vi "scanclass_1ms_10dt.vi"() -> (0 "max jitter (uS)":dbl format="%.2f", 1 "mean time (uS)":dbl format="%.2f", 2 "standard deviation (uS)":dbl format="%.2f", 3 "execution histogram":T1(graph), 4 "Error":errorcluster, 5 "execution times (uS)":dbl[](graph))   [LabVIEW 2013]
uses:
  scan engine timing source/scan engine timing source.lvclass
  scan engine timing source/scan engine timing source.lvclass/scan engine timing source.ctl
  <vilib>/Platform/TimedLoop/XDataNode/timing_clust.ctl
  <vilib>/Platform/TimedLoop/XDataNode/nitl_modes.ctl
  <vilib>/Platform/TimedLoop/XDataNode/wakeup.ctl
  scan engine timing source/Write scan period (uSec).vi
  <vilib>/platform/TimedLoop/XDataNode/XDataNode.xnode
  <vilib>/Platform/TimedLoop/XDataNode/XDNodeRunTimeDep.lvlib
  <vilib>/NI_Real-Time Target Support.lvlib
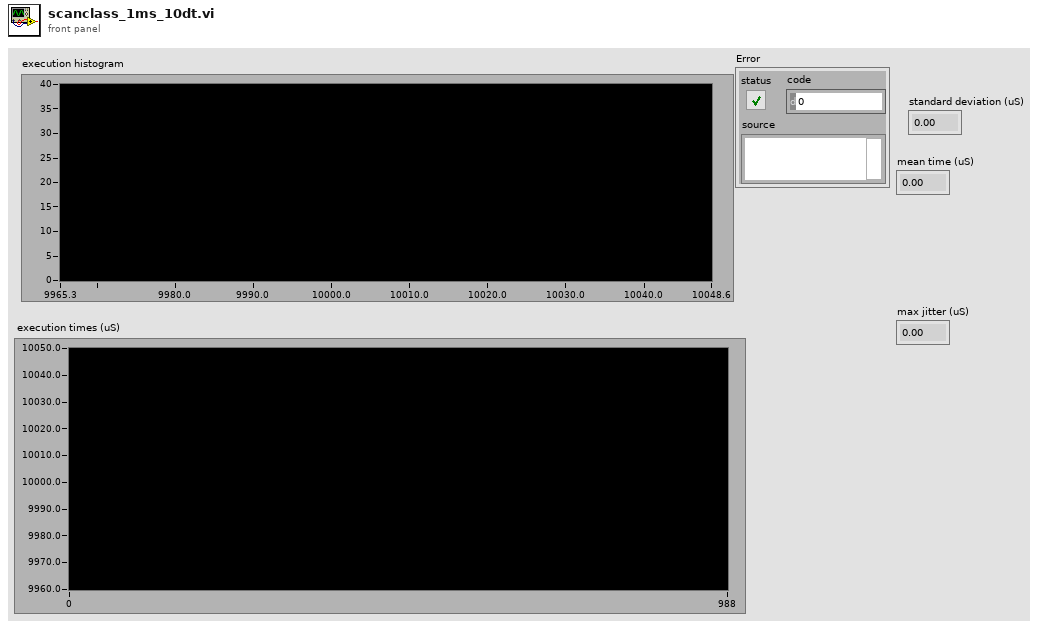
[diagram p1: front panel]
types:
  T1 = cluster{"X Values":dbl[], "Histogram: h(x)":i32[]}
  T2 = typedef "XDNodeRunTimeDep.lvlib/timing_clust.ctl" = cluster{"Expected End [f-1]":u64, "Actual End [f-1]":u64, "Finished Late? [f-1]":bool, "Expected End [i-1]":u64, "Actual End [i-1]":u64, "Finished Late? [i-1]":bool, "Expected Start [i]":u64, "Actual Start [i]":u64, "Expected Start [f]":u64, "Actual Start [f]":u64, "Source Name":string, "Structure Name":string, "Period":i64, "Deadline":i64, "Offset":i64, "Start":i64, "Priority":i32, "Timeout":i32, "Mode":T3, "Wakeup Reason":T4, "Error":errorcluster, "Source Type":string, "Secondary Source Type":string, "Global End Time":u64, "Global Start Time":u64, "Frame Duration":u64, "Iteration Duration":u64, "Assigned CPU":i32, "I/O Scan Engine Mode":u32}
  T3 = typedef "XDNodeRunTimeDep.lvlib/nitl_modes.ctl" = enum32{"No Change", "Process missed periods, maintain original phase", "Discard missed periods, maintain original phase", "Process missed periods, ignore original phase", "Discard missed periods, ignore original phase"}
  T4 = typedef "XDNodeRunTimeDep.lvlib/wakeup.ctl" = enum32{"Normal", "Aborted", "Asynchronous wakeup", "Timing source error", "Timed loop error", "Timeout"}
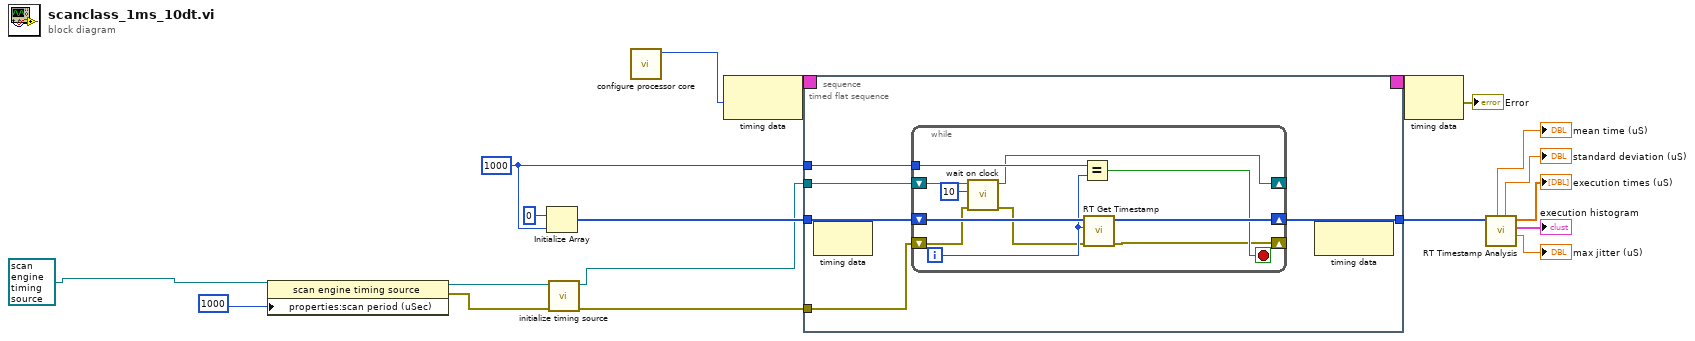
[diagram p0: block diagram]
diagram:
  w17 = 1000 ("x")
  n1 = property class="scan engine timing source"(reference=refnum<class "scan engine timing source.lvclass"> refnum ("scan engine timing source.lvclass"), "properties:scan period (uSec)"=u32 1000 ("scan period (uSec)")) -> (reference out=w5:refnum<class "scan engine timing source.lvclass">, error out=w3:errorcluster)  [unwired: 1 in]
  n2 = Initialize Array(u64 0, w17) -> (w18:u64[])
  n3 = call-dynamic "initialize timing source.vi"("error in"=w3, "timing source in"=w5) -> ("error out"=w1:errorcluster, "timing source out"=w2:refnum<class "scan engine timing source.lvclass">)  [unwired: 8 in]
  n4 = call "configure processor core.vi"() -> ("Processor"=w7:i32)  [unwired: 11 in]
  n5 = node-c288(w7) -> (w10:T2)
  n6 = timed-sequence {
    timing: w10 -> [_]
    timing-out: [_] -> w9
    tunnel: w17 -> [w24]
    tunnel: w18 -> [w23]
    tunnel: [w22] -> w16
    tunnel: w2 -> [w21]
    tunnel: w1 -> [w20]
    n7 = timed-flat-sequence {
      tunnel: w24 -> [w29]
      tunnel: w23 -> [w28]
      tunnel: [w27] -> w22
      tunnel: w21 -> [w26]
      tunnel: w20 -> [w25]
      n8 = node-c288() -> ()  [unwired: 1 in, 1 out]
      n9 = while {
        tunnel: w29 -> [w40]
        shift-right: [w38] -> w27
        shift-left: w28 -> [w39]
        shift-right: [w33] -> _
        shift-left: w26 -> [w34]
        shift-right: [w32] -> _
        shift-left: w25 -> [w31]
        i -> [w36]
        stop <- w37 stop-if-true
        n10 = call-dynamic "wait on clock.vi"("error in"=w31, "dt"=u32 10, "timing source in"=w34) -> ("error out"=w35:errorcluster, "timing source out"=w33:refnum<class "scan engine timing source.lvclass">)  [unwired: 6 in, 1 out]
        n11 = Equal?(x=w40, y=w36) -> (x = y?=w37:bool)
        n12 = call <vilib>:"RT Get Timestamp.vi"("error in (no error)"=w35, "iteration"=w36, "timestamp array in"=w39) -> ("error out"=w32:errorcluster, "timestamp array out"=w38:u64[])  [unwired: 7 in]
      }
      n13 = node-c288() -> ()  [unwired: 1 in, 1 out]
    }
  }
  n14 = node-c288(w9) -> (→"Error":errorcluster)
  n15 = call <vilib>:"RT Timestamp Analysis.vi"("timestamp array"=w16) -> ("max jitter (uS)"=→"max jitter (uS)":dbl, "execution histogram"=→"execution histogram":T1, "execution times (uS)"=→"execution times (uS)":dbl[], "standard deviation (uS)"=→"standard deviation (uS)":dbl, "mean time (uS)"=→"mean time (uS)":dbl)  [unwired: 5 in, 1 out]
